vi "Read From Symbol.vi"() -> ()   [LabVIEW 2018]
uses:
  47a29b1c-94e0-4f7c-b184-b17d399a3bf6.vi
  TwinCAT ADS Class/VIs/Data/Read.vi
  TwinCAT ADS Class/TwinCAT ADS.lvclass
panel:
  out "HTTP Request Messages":T1(array[cluster]) {"Request Line"."Method" items=["GET", "HEAD", "POST", "PUT", "DELETE", "CONNECT", "OPTIONS"]}
  # "Example PLC Source Code is available at:\nhttps://github.com/fisothemes/LabVIEW-TwinCAT-ADS/tree/master/src/PLC"
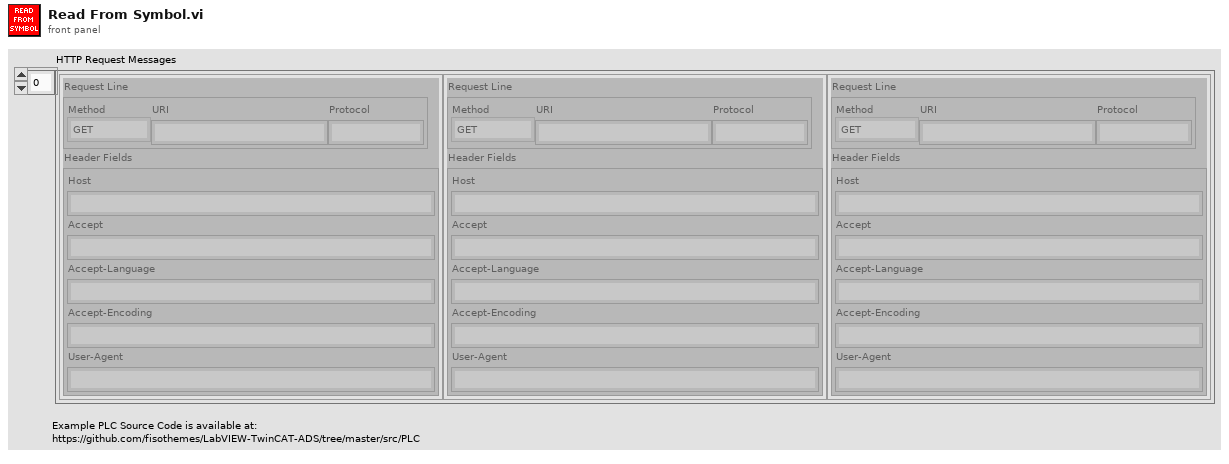
[diagram p1: front panel]
types:
  T1 = cluster{"Request Line":cluster{"Method":u16, "URI":string, "Protocol":string}, "Header Fields":cluster{"Host":string, "Accept":string, "Accept-Language":string, "Accept-Encoding":string, "User-Agent":string}}[]
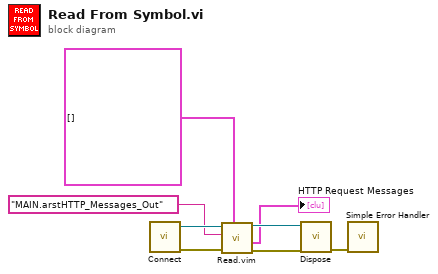
[diagram p0: block diagram]
diagram:
  n1 = call "Connect.vi"() -> ("error out"=w7:errorcluster, "TwinCAT ADS out"=w6:refnum<class "TwinCAT ADS.lvclass">)  [unwired: 10 in]
  n2 = call "Read.vim"("Type"=T1 [] ("HTTP Request Messages"), "error in (no error)"=w7, "Symbol Name"="MAIN.arstHTTP_Messages_Out" ("Name"), "TwinCAT ADS in"=w6) -> ("error out"=w3:errorcluster, "Value"=→"HTTP Request Messages":T1, "TwinCAT ADS out"=w2:refnum<class "TwinCAT ADS.lvclass">)  [unwired: 5 in]
  n3 = call "Dispose.vi"("error in (no error)"=w3, "TwinCAT ADS in"=w2) -> ("error out"=w8:errorcluster)  [unwired: 9 in]
  n4 = call <vilib>:"Simple Error Handler.vi"("error in (no error)"=w8) -> ()  [unwired: 4 in, 5 out]
